vi "单参数数据组装.vi"(9 "跨度值":dbl format="%#_13g", 10 "数据类别":u16(ring) items=["水样数据"=0, "标样数据"=1, "零点核查数据"=2, "跨度核查数据"=3, "环境变量"=4, "水样数据补传"=16, "标样核查数据补传"=17, "零点核查数据补传"=18, "跨度核查数据补传"=19], 11 "污染物":u16(ring)=1 items=["水温"=1, "浊度"=2, "DO"=3, "pH"=4, "ORP"=5, "比电导率"=6, "叶绿素a"=7, "氨氮"=8, "亚硝氮"=9, "硫化物"=10, "经度"=11, "维度"=12, "电压"=13]) -> (2 "data":T1 {"数据类别" items=["水样数据"=0, "标样数据"=1, "零点核查数据"=2, "跨度核查数据"=3, "环境变量"=4, "水样数据补传"=16, "标样核查数据补传"=17, "零点核查数据补传"=18, "跨度核查数据补传"=19]; "数组"."污染物" items=["水温"=1, "浊度"=2, "DO"=3, "pH"=4, "ORP"=5, "比电导率"=6, "叶绿素a"=7, "氨氮"=8, "亚硝氮"=9, "硫化物"=10, "电压"=11, "温度"=12, "湿度"=13, "GPS经度"=14, "GPS纬度"=15, "BD经度"=16, "BD纬度"=17]; "数组"."标识" items=["N"=1, "T"=2, "L"=3, "D"=4, "Z"=5, "M"=6, "hd"=7]}, 3 "布尔":bool)   [LabVIEW 2016, in "环境动力监测库.lvlib" / "NMEA.lvlib"]
uses:
  NMEA.lvlib
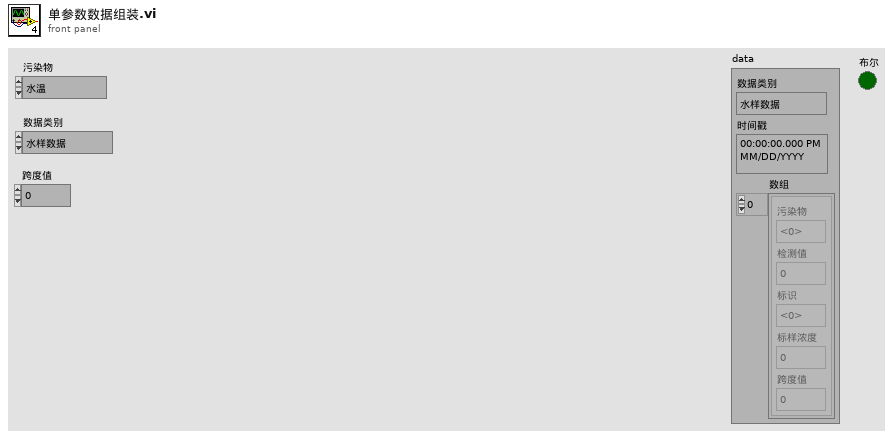
[diagram p1: front panel]
types:
  T1 = cluster{"数据类别":u16, "时间戳":timestamp, "数组":cluster{"污染物":u16, "检测值":dbl, "标识":u16, "标样浓度":dbl, "跨度值":dbl}[]}
  T2 = cluster{"时间标识":timestamp, "测量模式":string, "检测值":dbl, "数据标识":string, "标样参考值":dbl}[]
  T3 = cluster{"污染物":u16, "检测值":dbl, "标识":u16, "标样浓度":dbl, "跨度值":dbl}[]
  T4 = cluster{"数据类别":u16, "start time":timestamp, "数组":cluster{"污染物":u16, "检测值":dbl, "标识":u16, "标样浓度":dbl, "跨度值":dbl}[]}
  T5 = cluster{"时间标识":timestamp, "测量模式":string, "检测值":dbl, "数据标识":string, "标样参考值":dbl}
  T6 = cluster{"污染物":u16, "检测值":dbl, "标识":u16, "标样参考值":dbl, "跨度值":dbl}
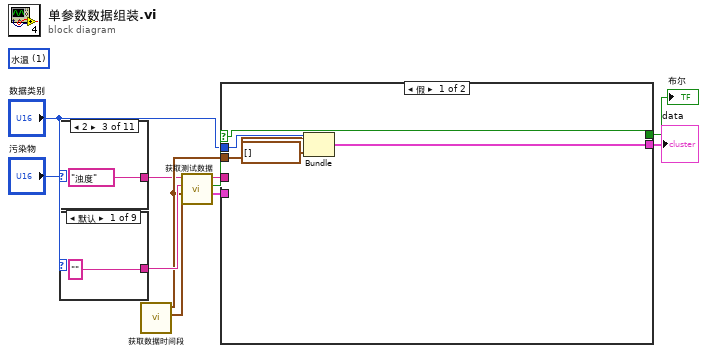
[diagram p0: block diagram]
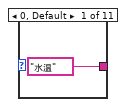
[diagram p2: hidden frame]
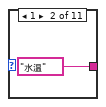
[diagram p3: hidden frame]
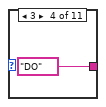
[diagram p4: hidden frame]
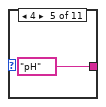
[diagram p5: hidden frame]
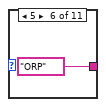
[diagram p6: hidden frame]
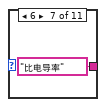
[diagram p7: hidden frame]
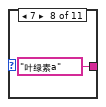
[diagram p8: hidden frame]
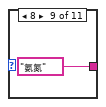
[diagram p9: hidden frame]
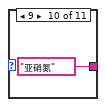
[diagram p10: hidden frame]
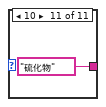
[diagram p11: hidden frame]
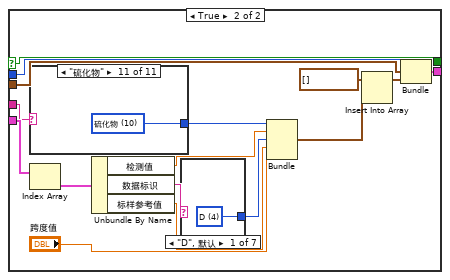
[diagram p12: hidden frame]
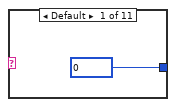
[diagram p13: hidden frame]
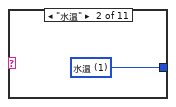
[diagram p14: hidden frame]
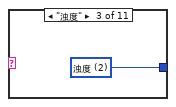
[diagram p15: hidden frame]
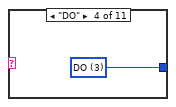
[diagram p16: hidden frame]
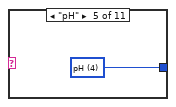
[diagram p17: hidden frame]
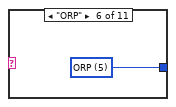
[diagram p18: hidden frame]
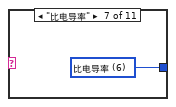
[diagram p19: hidden frame]
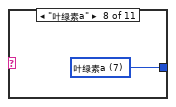
[diagram p20: hidden frame]
diagram:
  (unwired) u16 1 items=["水温"=1, "浊度"=2, "DO"=3, "pH"=4, "ORP"=5, "比电导率"=6, "叶绿素a"=7, "氨氮"=8, "亚硝氮"=9, "硫化物"=10, "电压"=11, "温度"=12, "湿度"=13, "GPS经度"=14, "GPS纬度"=15, "BD经度"=16, "BD纬度"=17] ("污染物")
  n1 = case shown="2" "污染物" {
    tunnel: ["水温" ("组合框") "水温" ("组合框") "浊度" ("组合框") "DO" ("组合框") "pH" ("组合框") "ORP" ("组合框") "比电导率" ("组合框") "叶绿素a" ("组合框") "氨氮" ("组合框") "亚硝氮" ("组合框") "硫化物" ("组合框")] -> w3
    frame 0, Default {
    }
    frame 1 {
    }
    frame 2 {
    }
    frame 3 {
    }
    frame 4 {
    }
    frame 5 {
    }
    frame 6 {
    }
    frame 7 {
    }
    frame 8 {
    }
    frame 9 {
    }
    frame 10 {
    }
  }
  n2 = case shown="默认" "数据类别" {
    tunnel: ["" ("组合框") "水样测试" ("组合框") "标样核查" ("组合框") "零点核查" ("组合框") "跨度核查" ("组合框") "水样测试" ("组合框") "标样核查" ("组合框") "零点核查" ("组合框") "跨度核查" ("组合框")] -> w8
    frame Default {
    }
    frame 0 {
    }
    frame 1 {
    }
    frame 2 {
    }
    frame 3 {
    }
    frame 16 {
    }
    frame 17 {
    }
    frame 18 {
    }
    frame 19 {
    }
  }
  n3 = call "获取数据时间段.vi"() -> ("end time"=w11:timestamp, "start time"=w7:timestamp)  [unwired: 10 in]
  n4 = call "获取测试数据.vi"("end time"=w11, "start time"=w7, "测量模式"=w8, "table"=w3) -> ("data"=w10:T2, "有数据"=w6:bool, "table 2"=w9:string)  [unwired: 5 in]
  n5 = case shown="假" w6 {
    selector: w6 -> [w36 w38]
    tunnel: w10 -> [_ w50]
    tunnel: w9 -> [_ w49]
    tunnel: "数据类别" -> [w35 w42]
    tunnel: w7 -> [w33 w41]
    tunnel: [w34 w39] -> w1
    tunnel: [w36 w38] -> w5
    frame False {
      n6 = Bundle("数据类别"=w35, "start time"=w33, "数组"=T3 []) -> (w34:T4)  [unwired: 1 in]
    }
    frame True {
      n7 = case shown="\"硫化物\"" w49 {
        tunnel: [w53 w54 w55 w56 w57 w58 w59 w60 w61 w62 w63] -> w48
        frame Default {
          w53 = u16 0 items=["水温"=1, "浊度"=2, "DO"=3, "pH"=4, "ORP"=5, "比电导率"=6, "叶绿素a"=7, "氨氮"=8, "亚硝氮"=9, "硫化物"=10, "电压"=11, "温度"=12, "湿度"=13, "GPS经度"=14, "GPS纬度"=15, "BD经度"=16, "BD纬度"=17] ("污染物")
        }
        frame "水温" {
          w54 = u16 1 items=["水温"=1, "浊度"=2, "DO"=3, "pH"=4, "ORP"=5, "比电导率"=6, "叶绿素a"=7, "氨氮"=8, "亚硝氮"=9, "硫化物"=10, "电压"=11, "温度"=12, "湿度"=13, "GPS经度"=14, "GPS纬度"=15, "BD经度"=16, "BD纬度"=17] ("污染物")
        }
        frame "浊度" {
          w55 = u16 2 items=["水温"=1, "浊度"=2, "DO"=3, "pH"=4, "ORP"=5, "比电导率"=6, "叶绿素a"=7, "氨氮"=8, "亚硝氮"=9, "硫化物"=10, "电压"=11, "温度"=12, "湿度"=13, "GPS经度"=14, "GPS纬度"=15, "BD经度"=16, "BD纬度"=17] ("污染物")
        }
        frame "DO" {
          w56 = u16 3 items=["水温"=1, "浊度"=2, "DO"=3, "pH"=4, "ORP"=5, "比电导率"=6, "叶绿素a"=7, "氨氮"=8, "亚硝氮"=9, "硫化物"=10, "电压"=11, "温度"=12, "湿度"=13, "GPS经度"=14, "GPS纬度"=15, "BD经度"=16, "BD纬度"=17] ("污染物")
        }
        frame "pH" {
          w57 = u16 4 items=["水温"=1, "浊度"=2, "DO"=3, "pH"=4, "ORP"=5, "比电导率"=6, "叶绿素a"=7, "氨氮"=8, "亚硝氮"=9, "硫化物"=10, "电压"=11, "温度"=12, "湿度"=13, "GPS经度"=14, "GPS纬度"=15, "BD经度"=16, "BD纬度"=17] ("污染物")
        }
        frame "ORP" {
          w58 = u16 5 items=["水温"=1, "浊度"=2, "DO"=3, "pH"=4, "ORP"=5, "比电导率"=6, "叶绿素a"=7, "氨氮"=8, "亚硝氮"=9, "硫化物"=10, "电压"=11, "温度"=12, "湿度"=13, "GPS经度"=14, "GPS纬度"=15, "BD经度"=16, "BD纬度"=17] ("污染物")
        }
        frame "比电导率" {
          w59 = u16 6 items=["水温"=1, "浊度"=2, "DO"=3, "pH"=4, "ORP"=5, "比电导率"=6, "叶绿素a"=7, "氨氮"=8, "亚硝氮"=9, "硫化物"=10, "电压"=11, "温度"=12, "湿度"=13, "GPS经度"=14, "GPS纬度"=15, "BD经度"=16, "BD纬度"=17] ("污染物")
        }
        frame "叶绿素a" {
          w60 = u16 7 items=["水温"=1, "浊度"=2, "DO"=3, "pH"=4, "ORP"=5, "比电导率"=6, "叶绿素a"=7, "氨氮"=8, "亚硝氮"=9, "硫化物"=10, "电压"=11, "温度"=12, "湿度"=13, "GPS经度"=14, "GPS纬度"=15, "BD经度"=16, "BD纬度"=17] ("污染物")
        }
        frame "氨氮" {
          w61 = u16 8 items=["水温"=1, "浊度"=2, "DO"=3, "pH"=4, "ORP"=5, "比电导率"=6, "叶绿素a"=7, "氨氮"=8, "亚硝氮"=9, "硫化物"=10, "电压"=11, "温度"=12, "湿度"=13, "GPS经度"=14, "GPS纬度"=15, "BD经度"=16, "BD纬度"=17] ("污染物")
        }
        frame "亚硝氮" {
          w62 = u16 9 items=["水温"=1, "浊度"=2, "DO"=3, "pH"=4, "ORP"=5, "比电导率"=6, "叶绿素a"=7, "氨氮"=8, "亚硝氮"=9, "硫化物"=10, "电压"=11, "温度"=12, "湿度"=13, "GPS经度"=14, "GPS纬度"=15, "BD经度"=16, "BD纬度"=17] ("污染物")
        }
        frame "硫化物" {
          w63 = u16 10 items=["水温"=1, "浊度"=2, "DO"=3, "pH"=4, "ORP"=5, "比电导率"=6, "叶绿素a"=7, "氨氮"=8, "亚硝氮"=9, "硫化物"=10, "电压"=11, "温度"=12, "湿度"=13, "GPS经度"=14, "GPS纬度"=15, "BD经度"=16, "BD纬度"=17] ("污染物")
        }
      }
      n8 = Index Array(array=w50) -> (element=w52:T5)  [unwired: 1 in]
      n9 = Unbundle By Name(w52) -> ("检测值"=w47:dbl, "数据标识"=w51:string, "标样参考值"=w37:dbl)
      n10 = case shown="\"D\", 默认" w51 {
        tunnel: [w64 w65 w66 w67 w68 w69 w70] -> w46
        frame "D", Default {
          w64 = u16 4 items=["N"=1, "T"=2, "L"=3, "D"=4, "Z"=5, "M"=6, "hd"=7] ("标识")
        }
        frame "N" {
          w65 = u16 1 items=["N"=1, "T"=2, "L"=3, "D"=4, "Z"=5, "M"=6, "hd"=7] ("标识")
        }
        frame "T" {
          w66 = u16 2 items=["N"=1, "T"=2, "L"=3, "D"=4, "Z"=5, "M"=6, "hd"=7] ("标识")
        }
        frame "L" {
          w67 = u16 3 items=["N"=1, "T"=2, "L"=3, "D"=4, "Z"=5, "M"=6, "hd"=7] ("标识")
        }
        frame "Z" {
          w68 = u16 5 items=["N"=1, "T"=2, "L"=3, "D"=4, "Z"=5, "M"=6, "hd"=7] ("标识")
        }
        frame "M" {
          w69 = u16 6 items=["N"=1, "T"=2, "L"=3, "D"=4, "Z"=5, "M"=6, "hd"=7] ("标识")
        }
        frame "hd" {
          w70 = u16 7 items=["N"=1, "T"=2, "L"=3, "D"=4, "Z"=5, "M"=6, "hd"=7] ("标识")
        }
      }
      n11 = Bundle("污染物"=w48, "检测值"=w47, "标识"=w46, "标样参考值"=w37, "跨度值"="跨度值") -> (w44:T6)  [unwired: 1 in]
      n12 = Insert Into Array(array=T3 [] ("数组"), new element=w44) -> (w40:T3)  [unwired: 1 in]
      n13 = Bundle("数据类别"=w42, "start time"=w41, "数组"=w40) -> (w39:T4)  [unwired: 1 in]
    }
  }
  "布尔" <- w5
  "data" <- w1
